vi "Initialize.vi"(8 "error in":errorcluster, 11 "transmission data unit in":refnum<class "Transmission Data Unit.lvclass">) -> (0 "error out":errorcluster, 3 "transmission data unit out":refnum<class "Transmission Data Unit.lvclass">)   [LabVIEW 2021, in "Transmission Data Unit.lvclass"]
doc: "This method reads data off of the chosen bus and attempts to return a modbus modbus data unit in the alotted time."
uses:
  Transmission Data Unit.lvclass
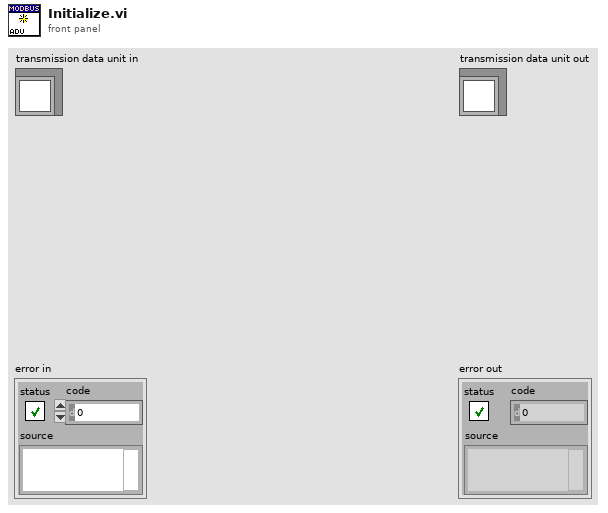
[diagram p1: front panel]
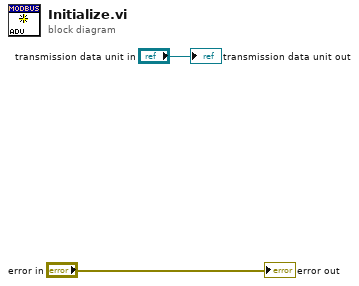
[diagram p0: block diagram]
diagram:
  "error out" <- "error in"
  "transmission data unit out" <- "transmission data unit in"
